vi "START.vi"() -> ()   [LabVIEW 2021]
uses:
  <vilib>/Instr/_visa.llb/VISA Configure Serial Port (Instr).vi
panel:
  in  "output":bool
  in  "set":bool
  in  "parity (0:none)":enum16{"None", "Odd", "Even", "Mark", "Space"}(ring)
  out "read_com_idn":string
  in  "connect_btn":bool
  out "read_com_string":string
  in  "read_from_com":bool
  in  "Current":dbl(knob) scale=0.0..4.0 scale format="%^#.3g"
  in  "Voltage":dbl(knob) scale=0.0..30.0 scale format="%^#.2g"
  in  "write buffer":string
  in  "write_to_com":bool
  in  "baud rate (9600)":u32=9600
  in  "VISA resource name":refnum<visa-resource-name>
  in  "stop":bool
  out "Waveform Chart":dbl(graph)
  out "daq_data":dbl
  # "TEMPERATURA Z TERMOPARY"
  # "POWER SUPPLY"
  # "COM-port:"
  # "Baud rate:"
  # "Parity:"
  # "SUPPLY ID:"
  # "WRITE COMMAND"
  # "READ CURRENT SETTINGS"
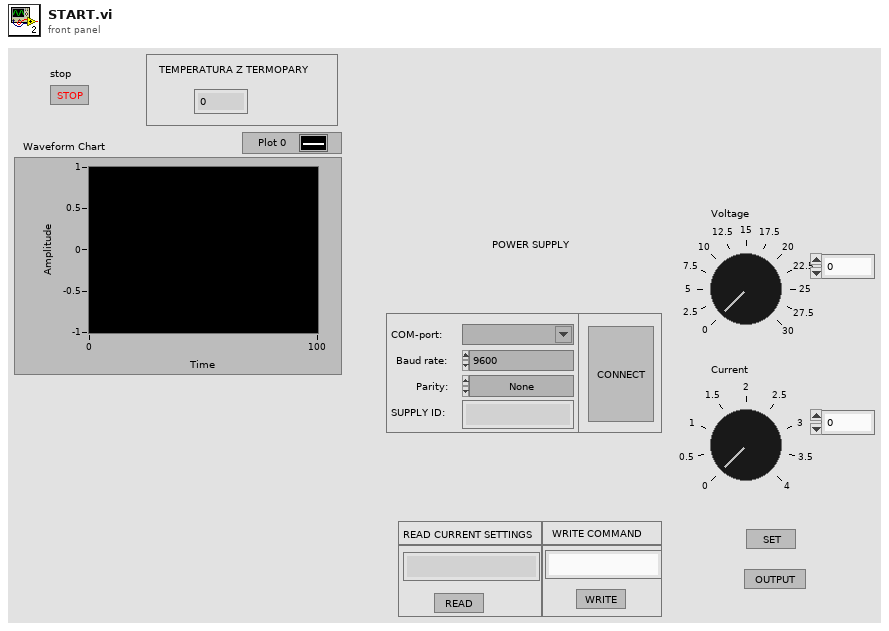
[diagram p1: front panel]
types:
  T1 = cluster{"daq_data":dbl, "COM_name":refnum<visa-resource-name>, "COM_baud":u32, "COM_parity":enum16{"None", "Odd", "Even", "Mark", "Space"}, "voltage_knob_value":dbl, "current_knob_value":dbl, "voltage_value_string":string, "current_value_string":string, "output_on_off":bool}
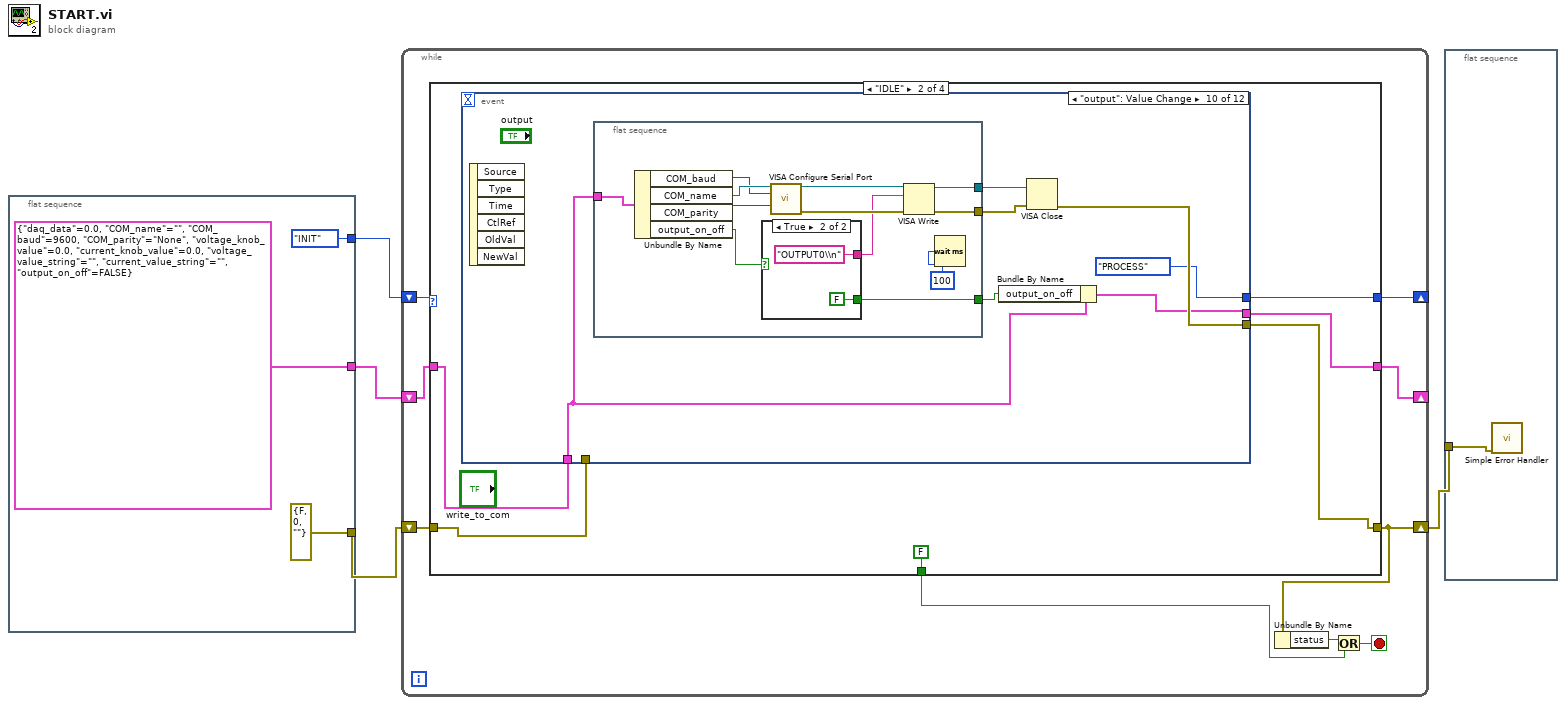
[diagram p0: block diagram]
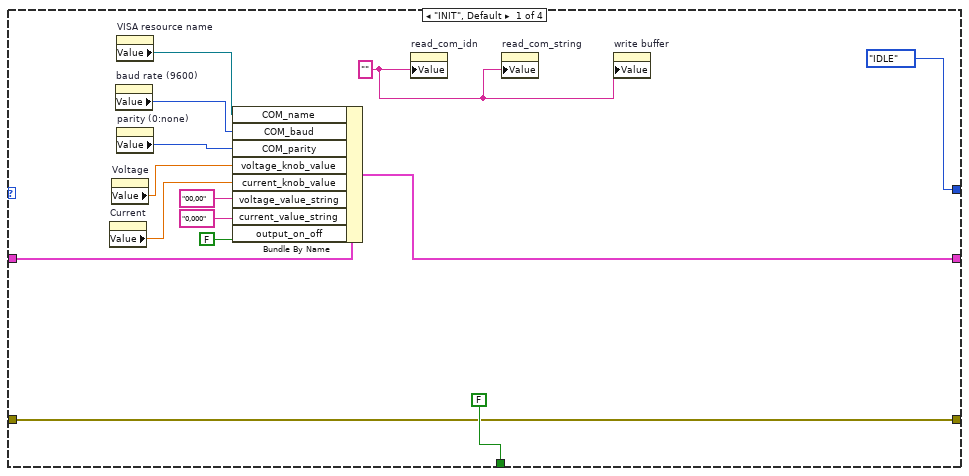
[diagram p2: hidden frame]
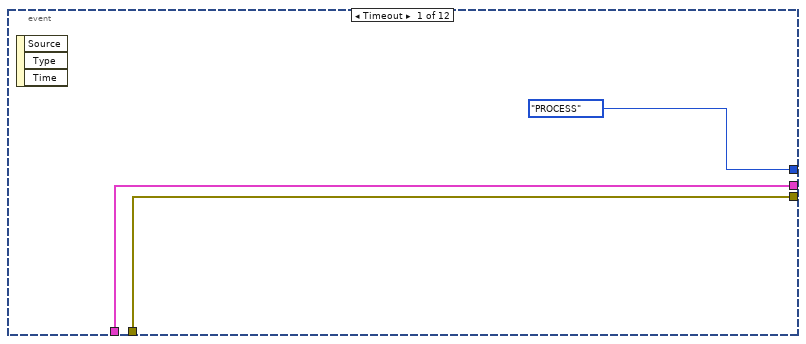
[diagram p3: hidden frame]
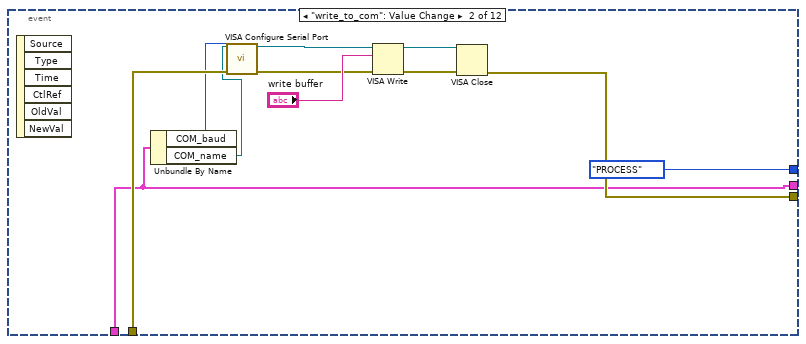
[diagram p4: hidden frame]
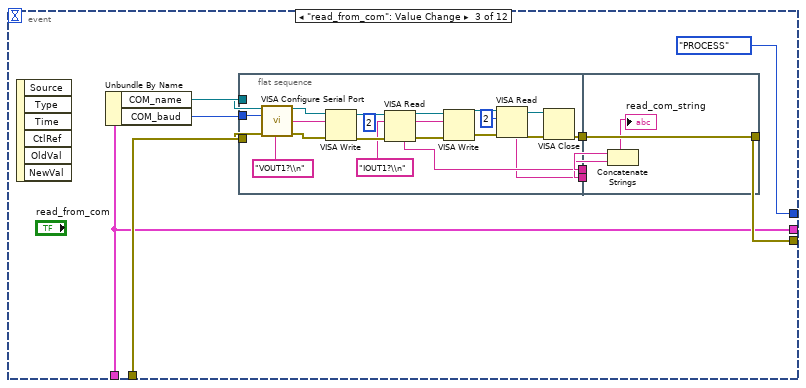
[diagram p5: hidden frame]
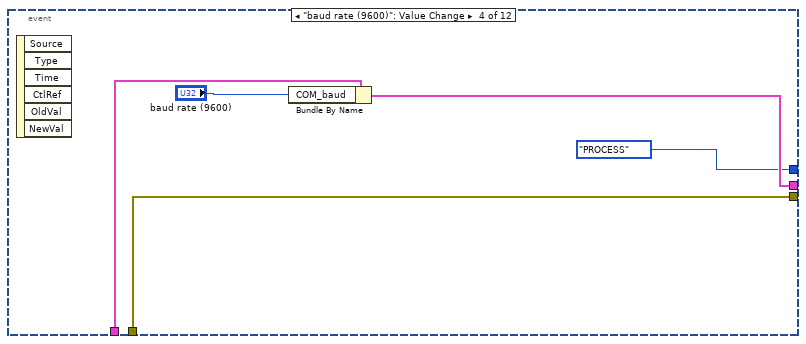
[diagram p6: hidden frame]
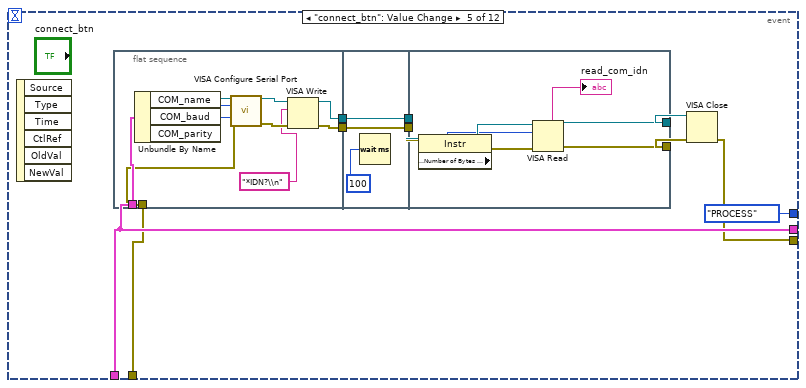
[diagram p7: hidden frame]
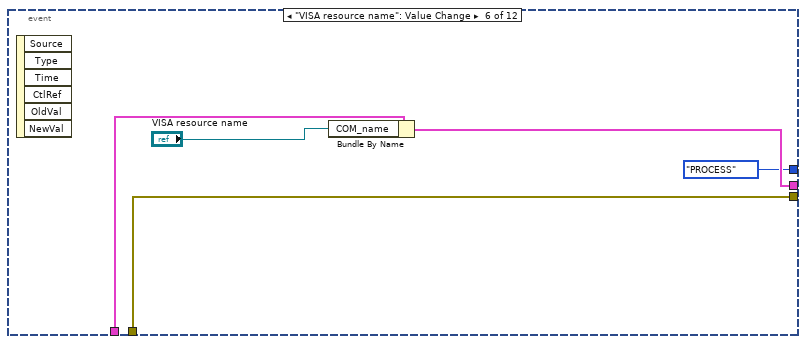
[diagram p8: hidden frame]
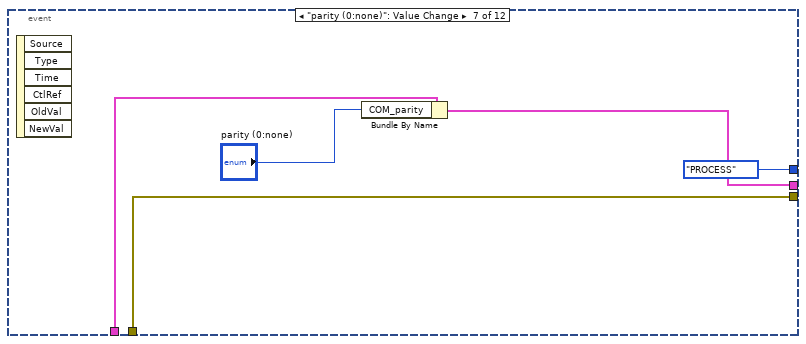
[diagram p9: hidden frame]
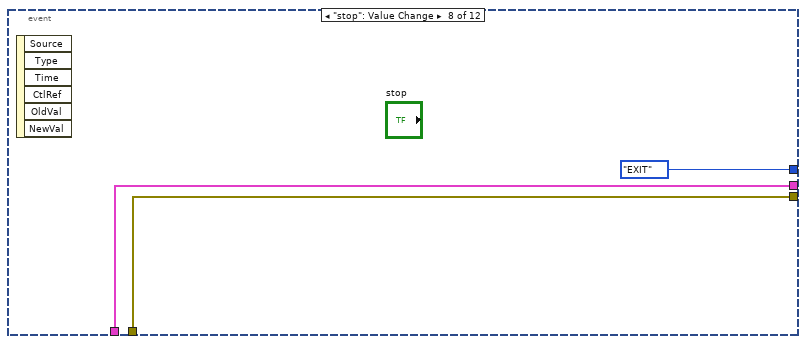
[diagram p10: hidden frame]
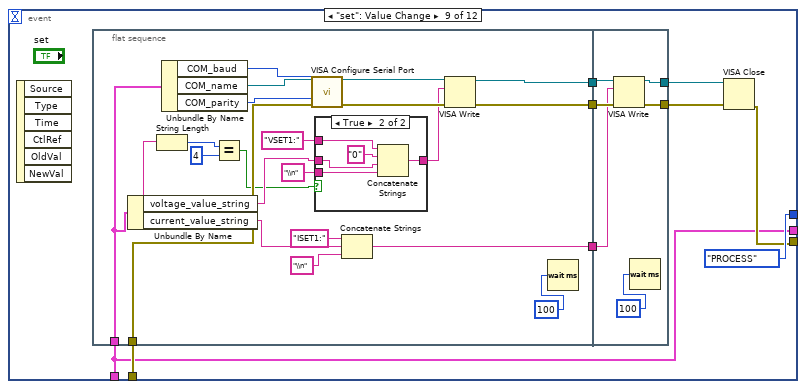
[diagram p11: hidden frame]
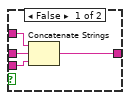
[diagram p12: hidden frame]
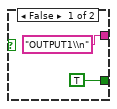
[diagram p13: hidden frame]
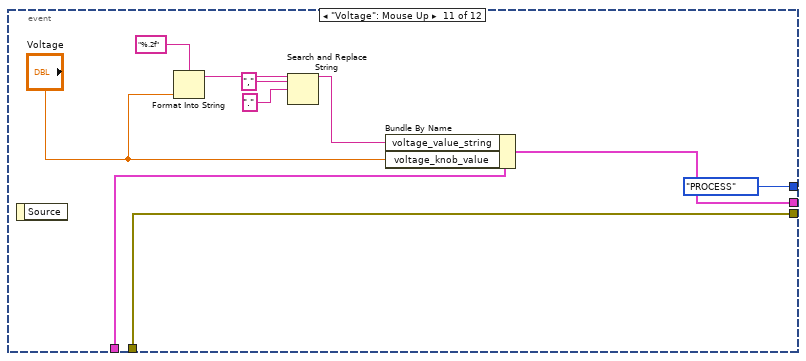
[diagram p14: hidden frame]
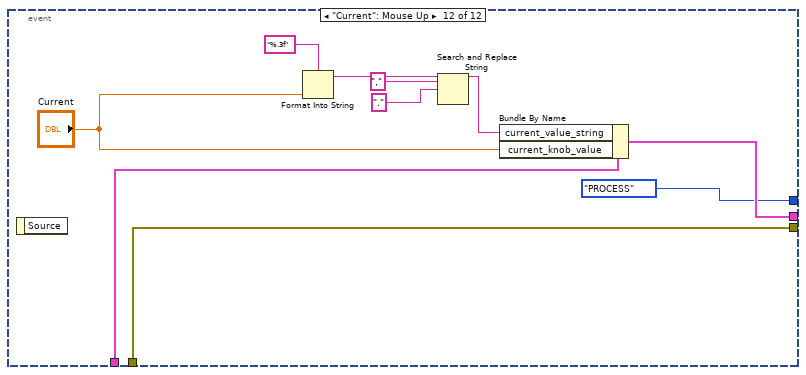
[diagram p15: hidden frame]
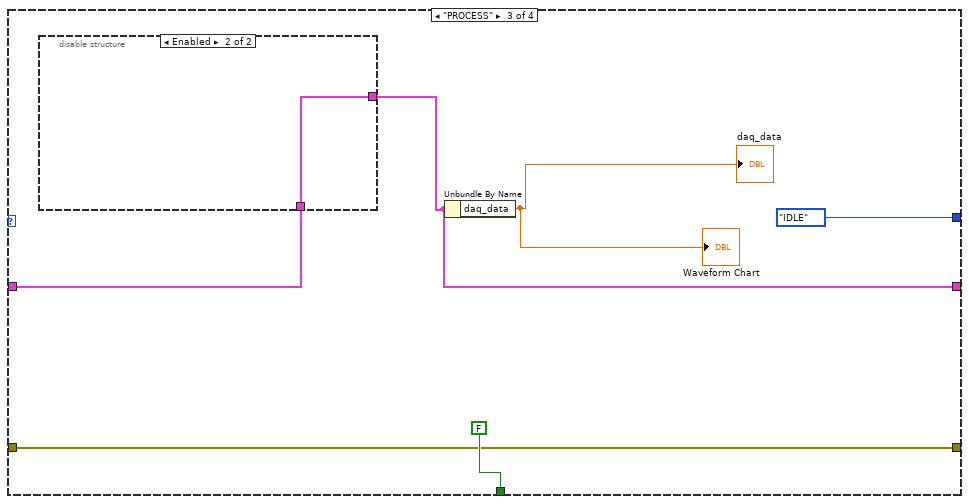
[diagram p16: hidden frame]
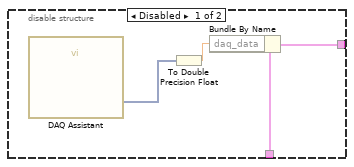
[diagram p17: hidden frame]
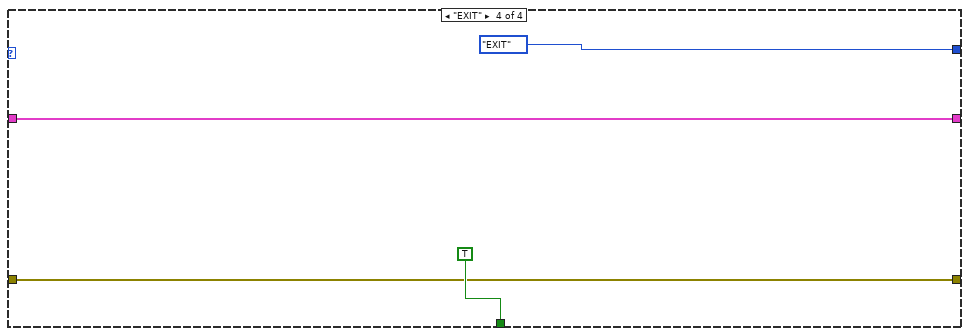
[diagram p18: hidden frame]
diagram:
  n1 = flat-sequence {
    tunnel: [enum16{"INIT", "IDLE", "PROCESS", "EXIT"}."INIT"] -> w4
    tunnel: [T1 {"daq_data"=0.0, "COM_name"="", "COM_baud"=9600, "COM_parity"=enum."None", "voltage_knob_value"=0.0, "current_knob_value"=0.0, "voltage_value_string"="", "current_value_string"="", "output_on_off"=FALSE}] -> w1
    tunnel: [errorcluster {"status"=FALSE, "code"=0, "source"=""} ("error in (no error)")] -> w2
    frame #0 {
    }
  }
  n2 = while {
    shift-right: [w15] -> _
    shift-left: w4 -> [w16]
    shift-right: [w14] -> _
    shift-left: w1 -> [w8]
    shift-right: [w11] -> w3
    shift-left: w2 -> [w12]
    stop <- w13 stop-if-true
    n3 = case shown="\"IDLE\"" w16 {
      tunnel: [FALSE FALSE FALSE TRUE] -> w9
      tunnel: [enum16{"INIT", "IDLE", "PROCESS", "EXIT"}."IDLE" w35 enum16{"INIT", "IDLE", "PROCESS", "EXIT"}."IDLE" enum16{"INIT", "IDLE", "PROCESS", "EXIT"}."EXIT"] -> w15
      tunnel: w8 -> [w25 w31 w222 w232]
      tunnel: [w24 w34 w221 w232] -> w14
      tunnel: w12 -> [w28 w33 w224 w233]
      tunnel: [w28 w32 w224 w233] -> w11
      frame "INIT", Default {
        w22 = "" ("read_com_idn")
        n4 = property on="Current" class="Knob (strict)"() -> ("Value"=w20:dbl)  [unwired: 2 in, 2 out]
        n5 = property on="Voltage" class="Knob (strict)"() -> ("Value"=w21:dbl)  [unwired: 2 in, 2 out]
        n6 = property on="baud rate (9600)" class="DigNum (strict)"() -> ("Value"=w27:u32)  [unwired: 2 in, 2 out]
        n7 = property on="VISA resource name" class="VISAName"() -> ("Value"=w26:refnum<visa-resource-name>)  [unwired: 2 in, 2 out]
        n8 = property on="parity (0:none)" class="Enum (strict)"() -> ("Value"=w23:enum16{"None", "Odd", "Even", "Mark", "Space"})  [unwired: 2 in, 2 out]
        n9 = Bundle By Name(cluster=w25, "COM_name"=w26, "COM_baud"=w27, "COM_parity"=w23, "voltage_knob_value"=w21, "current_knob_value"=w20, "voltage_value_string"="00,00", "current_value_string"="0,000" ("voltage_value_string"), "output_on_off"=FALSE) -> (w24:T1)
        n10 = property on="read_com_idn" class="Str"("Value"=w22) -> ()  [unwired: 2 in, 2 out]
        n11 = property on="read_com_string" class="Str"("Value"=w22) -> ()  [unwired: 2 in, 2 out]
        n12 = property on="write buffer" class="Str"("Value"=w22) -> ()  [unwired: 2 in, 2 out]
      }
      frame "IDLE" {
        n13 = event shown="[9] \"output\": Value Change" {
          selector: _ -> [_ _ _ _ _ _ _ _ _ _ _ _]
          dyn-events: _ -> [_ _ _ _ _ _ _ _ _ _ _ _]
          timeout: _ -> [_ _ _ _ _ _ _ _ _ _ _ _]
          tunnel: [enum16{"INIT", "IDLE", "PROCESS", "EXIT"}."PROCESS" enum16{"INIT", "IDLE", "PROCESS", "EXIT"}."PROCESS" enum16{"INIT", "IDLE", "PROCESS", "EXIT"}."PROCESS" enum16{"INIT", "IDLE", "PROCESS", "EXIT"}."PROCESS" enum16{"INIT", "IDLE", "PROCESS", "EXIT"}."PROCESS" enum16{"INIT", "IDLE", "PROCESS", "EXIT"}."PROCESS" enum16{"INIT", "IDLE", "PROCESS", "EXIT"}."PROCESS" enum16{"INIT", "IDLE", "PROCESS", "EXIT"}."EXIT" enum16{"INIT", "IDLE", "PROCESS", "EXIT"}."PROCESS" enum16{"INIT", "IDLE", "PROCESS", "EXIT"}."PROCESS" enum16{"INIT", "IDLE", "PROCESS", "EXIT"}."PROCESS" enum16{"INIT", "IDLE", "PROCESS", "EXIT"}."PROCESS"] -> w35
          tunnel: [w38 w42 w53 w87 w97 w123 w127 w131 w137 w179 w209 w219] -> w34
          tunnel: w31 -> [w38 w42 w53 w88 w97 w124 w129 w131 w137 w180 w210 w220]
          tunnel: w33 -> [w37 w46 w59 w84 w96 w121 w125 w130 w139 _ w207 w218]
          tunnel: [w37 w43 w58 w84 w95 w121 w125 w130 w138 w182 w207 w218] -> w32
          event Timeout {
            n14 = event-data() -> ()  [unwired: 1 in, 3 out]
          }
          event "write_to_com": Value Change {
            n15 = event-data() -> ()  [unwired: 1 in, 6 out]
            n16 = Unbundle By Name(w42) -> ("COM_baud"=w41:u32, "COM_name"=w40:refnum<visa-resource-name>)
            n17 = call-poly "VISA Configure Serial Port"("VISA resource name"=w40, "baud rate (9600)"=w41, "error in (no error)"=w46) -> ("VISA resource name out"=w49:refnum<visa-resource-name>, "error out"=w45:errorcluster)  [unwired: 11 in]
            n18 = VISA Write(VISA resource name=w49, write buffer="write buffer", error in (no error)=w45) -> (VISA resource name out=w48:refnum<visa-resource-name>, error out=w44:errorcluster)  [unwired: 1 out]
            n19 = VISA Close(VISA resource name=w48, error in (no error)=w44) -> (error out=w43:errorcluster)
          }
          event "read_from_com": Value Change {
            n20 = event-data() -> ()  [unwired: 1 in, 6 out]
            n21 = Unbundle By Name(w53) -> ("COM_name"=w52:refnum<visa-resource-name>, "COM_baud"=w51:u32)
            n22 = flat-sequence {
              tunnel: w59 -> [w79]
              tunnel: [w78] -> w56
              tunnel: [w65] -> w55
              tunnel: [w64] -> w54
              tunnel: w52 -> [w61]
              tunnel: w51 -> [w60]
              tunnel: [w83] -> w58
              tunnel: w56 -> [w83]
              tunnel: w55 -> [w81]
              tunnel: w54 -> [w80]
              frame #0 {
                n23 = call-poly "VISA Configure Serial Port"("VISA resource name"=w61, "baud rate (9600)"=w60, "error in (no error)"=w79) -> ("VISA resource name out"=w77:refnum<visa-resource-name>, "error out"=w75:errorcluster)  [unwired: 11 in]
                n24 = VISA Write(VISA resource name=w77, write buffer="VOUT1?\\n", error in (no error)=w75) -> (VISA resource name out=w76:refnum<visa-resource-name>, error out=w74:errorcluster)  [unwired: 1 out]
                n25 = VISA Read(VISA resource name=w76, byte count=u32 2, error in (no error)=w74) -> (VISA resource name out=w66:refnum<visa-resource-name>, read buffer=w65:string, error out=w67:errorcluster)  [unwired: 1 out]
                n26 = VISA Write(VISA resource name=w66, write buffer="IOUT1?\\n", error in (no error)=w67) -> (VISA resource name out=w70:refnum<visa-resource-name>, error out=w71:errorcluster)  [unwired: 1 out]
                n27 = VISA Read(VISA resource name=w70, byte count=u32 2, error in (no error)=w71) -> (VISA resource name out=w68:refnum<visa-resource-name>, read buffer=w64:string, error out=w69:errorcluster)  [unwired: 1 out]
                n28 = VISA Close(VISA resource name=w68, error in (no error)=w69) -> (error out=w78:errorcluster)
              }
              frame #1 {
                n29 = Concatenate Strings(w81, w80) -> (→"read_com_string":string)
              }
            }
          }
          event "baud rate (9600)": Value Change {
            n30 = event-data() -> ()  [unwired: 1 in, 6 out]
            n31 = Bundle By Name(cluster=w88, "COM_baud"="baud rate (9600)") -> (w87:T1)
          }
          event "connect_btn": Value Change {
            n32 = event-data() -> ()  [unwired: 1 in, 6 out]
            n33 = flat-sequence {
              tunnel: w97 -> [w103]
              tunnel: w96 -> [w102]
              tunnel: [w100] -> w92
              tunnel: [w99] -> w90
              tunnel: w92 -> [w111]
              tunnel: [w111] -> w91
              tunnel: w90 -> [w110]
              tunnel: [w110] -> w89
              tunnel: w91 -> [w115]
              tunnel: w89 -> [w114]
              tunnel: [w113] -> w94
              tunnel: [w112] -> w93
              frame #0 {
                n34 = Unbundle By Name(w103) -> ("COM_name"=w106:refnum<visa-resource-name>, "COM_baud"=w105:u32, "COM_parity"=w101:enum16{"None", "Odd", "Even", "Mark", "Space"})
                n35 = call-poly "VISA Configure Serial Port"("VISA resource name"=w106, "baud rate (9600)"=w105, "parity (0:none)"=w101, "error in (no error)"=w102) -> ("VISA resource name out"=w108:refnum<visa-resource-name>, "error out"=w107:errorcluster)  [unwired: 10 in]
                n36 = VISA Write(VISA resource name=w108, write buffer="*IDN?\\n", error in (no error)=w107) -> (VISA resource name out=w100:refnum<visa-resource-name>, error out=w99:errorcluster)  [unwired: 1 out]
              }
              frame #1 {
                n37 = Wait (ms)(milliseconds to wait=u32 100) -> ()  [unwired: 1 out]
              }
              frame #2 {
                n38 = property class="Instr"(reference=w115, error in=w114) -> (reference out=w118:refnum<visa-resource-name>, error out=w117:errorcluster, "Serial Settings:Number of Bytes at Serial Port"=w116:u32)
                n39 = VISA Read(VISA resource name=w118, byte count=w116, error in (no error)=w117) -> (VISA resource name out=w112:refnum<visa-resource-name>, read buffer=→"read_com_idn":string, error out=w113:errorcluster)  [unwired: 1 out]
              }
            }
            n40 = VISA Close(VISA resource name=w93, error in (no error)=w94) -> (error out=w95:errorcluster)
          }
          event "VISA resource name": Value Change {
            n41 = event-data() -> ()  [unwired: 1 in, 6 out]
            n42 = Bundle By Name(cluster=w124, "COM_name"="VISA resource name") -> (w123:T1)
          }
          event "parity (0:none)": Value Change {
            n43 = event-data() -> ()  [unwired: 1 in, 6 out]
            n44 = Bundle By Name(cluster=w129, "COM_parity"="parity (0:none)") -> (w127:T1)
          }
          event "stop": Value Change {
            n45 = event-data() -> ()  [unwired: 1 in, 6 out]
          }
          event "set": Value Change {
            n46 = event-data() -> ()  [unwired: 1 in, 6 out]
            n47 = flat-sequence {
              tunnel: w139 -> [w158]
              tunnel: w137 -> [w157]
              tunnel: [w161] -> w135
              tunnel: [w149] -> w134
              tunnel: [w143] -> w133
              tunnel: [w173] -> w136
              tunnel: [w172] -> w140
              tunnel: w135 -> [w176]
              tunnel: w134 -> [w175]
              tunnel: w133 -> [w174]
              frame #0 {
                n48 = Unbundle By Name(w157) -> ("voltage_value_string"=w155:string, "current_value_string"=w145:string)
                n49 = String Length(string=w155) -> (length=w154:i32)
                n50 = Unbundle By Name(w157) -> ("COM_baud"=w160:u32, "COM_name"=w159:refnum<visa-resource-name>, "COM_parity"=w156:enum16{"None", "Odd", "Even", "Mark", "Space"})
                n51 = Equal?(x=w154, y=4) -> (x = y?=w151:bool)
                n52 = call-poly "VISA Configure Serial Port"("VISA resource name"=w159, "baud rate (9600)"=w160, "parity (0:none)"=w156, "error in (no error)"=w158) -> ("VISA resource name out"=w148:refnum<visa-resource-name>, "error out"=w162:errorcluster)  [unwired: 10 in]
                n53 = case shown="True" w151 {
                  tunnel: [w166 w171] -> w147
                  tunnel: w155 -> [w164 w169]
                  tunnel: "VSET1:" ("string") -> [w165 w170]
                  tunnel: "\\n" ("string") -> [w163 w168]
                  frame False {
                    n54 = Concatenate Strings(w165, w164, w163) -> (w166:string)
                  }
                  frame True {
                    n55 = Concatenate Strings(w170, "0" ("string"), w169, w168) -> (w171:string)
                  }
                }
                n56 = Concatenate Strings("ISET1:" ("string"), w145, "\\n" ("string")) -> (w143:string)
                n57 = VISA Write(VISA resource name=w148, write buffer=w147, error in (no error)=w162) -> (VISA resource name out=w149:refnum<visa-resource-name>, error out=w161:errorcluster)  [unwired: 1 out]
                n58 = Wait (ms)(milliseconds to wait=u32 100) -> ()  [unwired: 1 out]
              }
              frame #1 {
                n59 = VISA Write(VISA resource name=w175, write buffer=w174, error in (no error)=w176) -> (VISA resource name out=w173:refnum<visa-resource-name>, error out=w172:errorcluster)  [unwired: 1 out]
                n60 = Wait (ms)(milliseconds to wait=u32 100) -> ()  [unwired: 1 out]
              }
            }
            n61 = VISA Close(VISA resource name=w136, error in (no error)=w140) -> (error out=w138:errorcluster)
          }
          event "output": Value Change {
            n62 = event-data() -> ()  [unwired: 1 in, 6 out]
            n63 = flat-sequence {
              tunnel: w180 -> [w193]
              tunnel: [w189] -> w184
              tunnel: [w188] -> w183
              tunnel: [w185] -> w178
              frame #0 {
                n64 = Unbundle By Name(w193) -> ("COM_baud"=w191:u32, "COM_name"=w192:refnum<visa-resource-name>, "COM_parity"=w190:enum16{"None", "Odd", "Even", "Mark", "Space"}, "output_on_off"=w186:bool)
                n65 = case shown="True" w186 {
                  tunnel: ["OUTPUT1\\n" ("write buffer") "OUTPUT0\\n" ("write buffer")] -> w187
                  tunnel: [TRUE FALSE] -> w185
                  frame False {
                  }
                  frame True {
                  }
                }
                n66 = call-poly "VISA Configure Serial Port"("VISA resource name"=w192, "baud rate (9600)"=w191, "parity (0:none)"=w190) -> ("VISA resource name out"=w195:refnum<visa-resource-name>, "error out"=w196:errorcluster)  [unwired: 11 in]
                n67 = VISA Write(VISA resource name=w195, write buffer=w187, error in (no error)=w196) -> (VISA resource name out=w189:refnum<visa-resource-name>, error out=w188:errorcluster)  [unwired: 1 out]
                n68 = Wait (ms)(milliseconds to wait=u32 100) -> ()  [unwired: 1 out]
              }
            }
            n69 = Bundle By Name(cluster=w180, "output_on_off"=w178) -> (w179:T1)
            n70 = VISA Close(VISA resource name=w184, error in (no error)=w183) -> (error out=w182:errorcluster)
          }
          event "Voltage": Mouse Up {
            n71 = event-data() -> ()  [unwired: 1 in, 1 out]
            n72 = Format Into String(format string="%.2f", "Voltage") -> (resulting string=w206:string)  [unwired: 2 in, 1 out]
            n73 = Search and Replace String(input string=w206, search string=",", replace string="." ("replace string (\"\")")) -> (result string=w201:string)  [unwired: 5 in, 3 out]
            n74 = Bundle By Name(cluster=w210, "voltage_value_string"=w201, "voltage_knob_value"="Voltage") -> (w209:T1)
          }
          event "Current": Mouse Up {
            n75 = event-data() -> ()  [unwired: 1 in, 1 out]
            n76 = Format Into String(format string="%.3f", "Current") -> (resulting string=w216:string)  [unwired: 2 in, 1 out]
            n77 = Search and Replace String(input string=w216, search string=",", replace string="." ("replace string (\"\")")) -> (result string=w211:string)  [unwired: 5 in, 3 out]
            n78 = Bundle By Name(cluster=w220, "current_value_string"=w211, "current_knob_value"="Current") -> (w219:T1)
          }
        }
      }
      frame "PROCESS" {
        n79 = disable-structure shown="Enabled" {
          disable-tunnel: w222 -> [w228 w231]
          disable-tunnel: [w227 w231] -> w221
          frame Disabled {
            n80 = call "DAQ Assistant"() -> ("data"=w229:dynamicdata)  [unwired: 17 in, 2 out]
            n81 = To Double Precision Float(number=w229) -> (double precision float=w230:dbl)
            n82 = Bundle By Name(cluster=w228, "daq_data"=w230) -> (w227:T1)
          }
          frame Enabled {
          }
        }
        n83 = Unbundle By Name(w221) -> ("daq_data"=→"daq_data" →"Waveform Chart":dbl)
      }
      frame "EXIT" {
      }
    }
    n84 = Unbundle By Name(w11) -> ("status"=w10:bool)
    n85 = Or(x=w10, y=w9) -> (x .or. y?=w13:bool)
  }
  n86 = flat-sequence {
    tunnel: w3 -> [w236]
    frame #0 {
      n87 = call <vilib>:"Simple Error Handler.vi"("error in (no error)"=w236) -> ()  [unwired: 4 in, 5 out]
    }
  }
